vi "ble_write_client_characterist_configuration.vi"(5 "Characteristic UUID":string, 6 "Connection Status":T1={"MAC Address"="", "cnx handle"=0, "cnx flags"=0, "Address Type"=125, "Connection Interval (ms)"=125, "Timeout(ms)"=125, "Latency"=0, "bonding handle"=0} {"Address Type" items=["Public", "Random"]}, 7 "Service UUID":string, 8 "error in (no error)":errorcluster, 9 "Value(16bit)":u16 format="%04x", 10 "Handle table":string[][](array[string]), 11 "COM Bluegiga in":refnum<visa-resource-name>) -> (0 "error out":errorcluster, 3 "COM Bluegiga out":refnum<visa-resource-name>)   [LabVIEW 2013]
uses:
  type_def/connection_status_bundle.ctl
  type_def/address_type.ctl
  ble_write_by_handle_uint16.vi
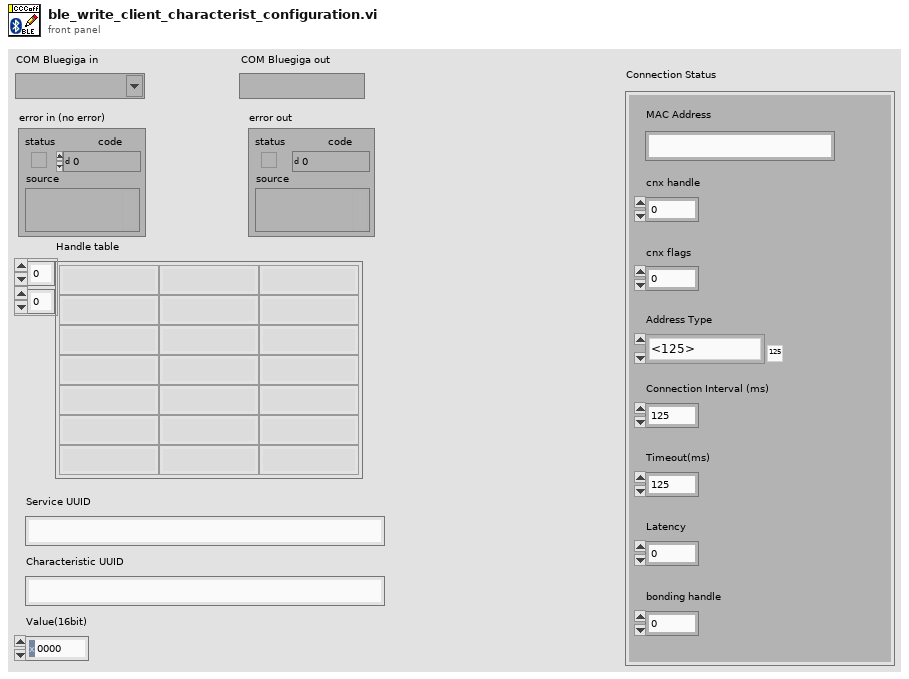
[diagram p1: front panel]
types:
  T1 = typedef "connection_status_bundle.ctl" = cluster{"MAC Address":string, "cnx handle":u8, "cnx flags":u8, "Address Type":T2, "Connection Interval (ms)":u16, "Timeout(ms)":u16, "Latency":u16, "bonding handle":u8}
  T2 = typedef "address_type.ctl" = u8
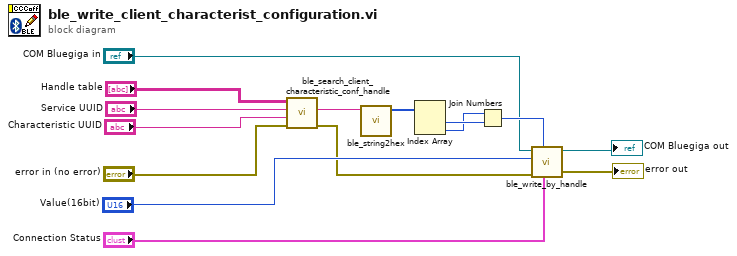
[diagram p0: block diagram]
diagram:
  n1 = call "ble_search_client_characteristic_conf_handle.vi"("error in (no error)"="error in (no error)", "Characteristic UUID"="Characteristic UUID", "Service UUID"="Service UUID", "Handle table"="Handle table") -> ("error out"=w5:errorcluster, "Handle"=w4:string)  [unwired: 6 in]
  n2 = call "ble_string2hex.vi"("HEX string IN"=w4) -> ("Byte Array IN (index0 LS byte)"=w11:u8[])  [unwired: 10 in]
  n3 = Index Array(array=w11) -> (element #1=w15:u8, element #2=w14:u8)  [unwired: 2 in]
  n4 = Join Numbers(hi=w14, lo=w15) -> ((hi.lo)=w3:u16)
  n5 = call-poly "ble_write_by_handle.vi"("Connection Status"="Connection Status", "Handle"=w3, "error in (no error)"=w5, "Value(uint16)"="Value(16bit)", "COM Bluegiga in"="COM Bluegiga in") -> ("error out"=→"error out":errorcluster, "COM Bluegiga out"=→"COM Bluegiga out":refnum<visa-resource-name>)  [unwired: 5 in]
